vi "Round SGL.vi"(11 "SGL":sgl) -> (3 "I32":i32)   [LabVIEW 2022 SP3, in "Raster.lvlib"]
doc: "Round the SGL to the nearest I32."
uses:
  Raster.lvlib
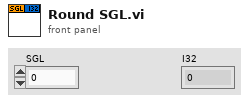
[diagram p1: front panel]
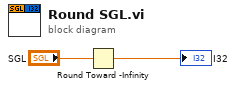
[diagram p0: block diagram]
diagram:
  n1 = Round Toward -Infinity(1:"SGL") -> (0:→"I32":sgl)
